vi "Wait on Notification.vi"(6 "timeout in ms (-1)":i32=-1, 8 "error in":errorcluster, 11 "NotifierMessageTransport in":refnum<class "NotifierMessageTransport.lvclass">) -> (0 "error out":errorcluster, 2 "Notification":refnum<class "IMessagePayload.lvclass">, 3 "NotifierMessageTransport out":refnum<class "NotifierMessageTransport.lvclass">)   [LabVIEW 2016, in "NotifierMessageTransport.lvclass"]
uses:
  NotifierMessageTransport.lvclass
  IMessagePayload/IMessagePayload.lvclass
  NotifierMessageTransport.lvclass/NotifierMessageTransport.ctl
panel:
  # "INPUTS"
  # "OUTPUTS"
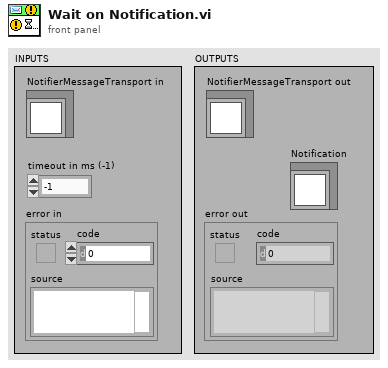
[diagram p1: front panel]
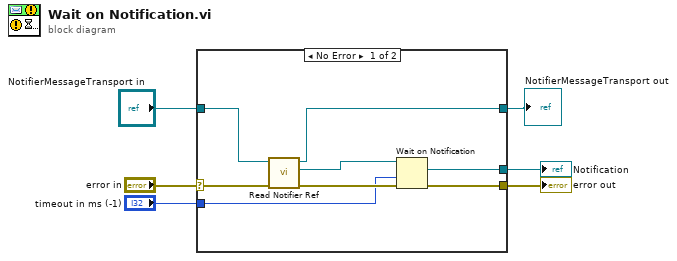
[diagram p0: block diagram]
diagram:
  n1 = case shown="No Error" "error in" {
    selector: "error in" -> [w14 w16]
    tunnel: [w8 w16] -> w5
    tunnel: [w12 w15] -> w3
    tunnel: "NotifierMessageTransport in" -> [w13 w15]
    tunnel: "timeout in ms (-1)" -> [w9 _]
    tunnel: [w7 _] -> w1
    frame No Error {
      n2 = call "Read Notifier Ref.vi"("error in"=w14, "NotifierMessageTransport in"=w13) -> ("error out"=w11:errorcluster, "Notifier Ref"=w10:refnum<notifier>, "NotifierMessageTransport out"=w12:refnum<class "NotifierMessageTransport.lvclass">)  [unwired: 7 in]
      n3 = Wait on Notification(notifier=w10, timeout in ms (-1)=w9, error in (no error)=w11) -> (notification=w7:refnum<class "IMessagePayload.lvclass">, error out=w8:errorcluster)  [unwired: 1 in, 2 out]
    }
    frame Error {
    }
  }
  "error out" <- w5
  "NotifierMessageTransport out" <- w3
  "Notification" <- w1
